vi "Controller.vi"() -> ()   [LabVIEW 2011]
panel:
  in  "Horizontal Pointer Slide":i32(slide) scale=0.0..10.0
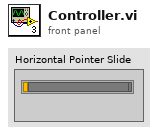
[diagram p1: front panel]
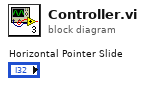
[diagram p0: block diagram]
diagram:
